vi "Build Type String.vi"(11 "Build in":refnum<class "Build.lvclass">) -> (2 "Build Type":string)   [LabVIEW 2020, in "Builder Tools.lvlib" / "Build.lvclass"]
uses:
  Build.lvclass
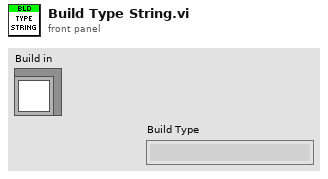
[diagram p1: front panel]
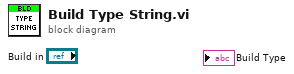
[diagram p0: block diagram]
diagram:
